vi "Get Test.vi"(8 "error in (no error)":errorcluster, 10 "Unique ID":string, 11 "Test Executive Ref":refnum<data-value>) -> (0 "error out":errorcluster, 1 "Found?":bool, 2 "Test":refnum<class "Executioner.lvclass">, 3 "Test Executive Ref out":refnum<data-value>)   [LabVIEW 2017, in "Test Executive.lvlib" / "TestExecutive Ref.lvclass"]
uses:
  <vilib>/gpm_packages/@cs/test-executive/Source/Test Executive/TestExecutive Ref/TestExecutive Ref.lvclass
  <vilib>/gpm_packages/@cs/test-executive/Source/Test Executive/ITestExecutive/ITest Executive.lvclass
  <vilib>/gpm_packages/@cs/test-executive/Source/Test Executive/Executioner/Executioner.lvclass
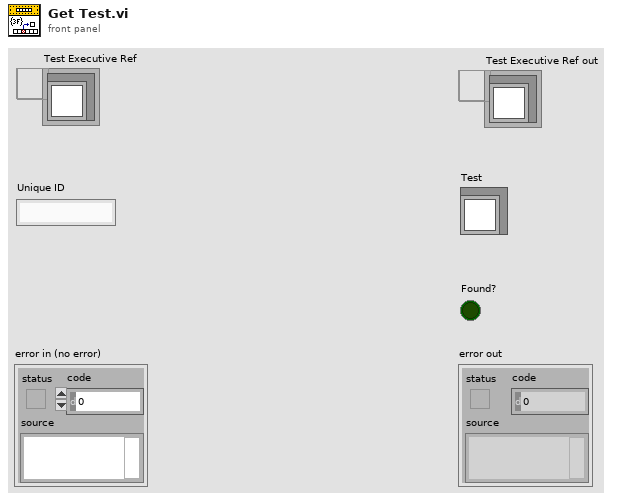
[diagram p1: front panel]
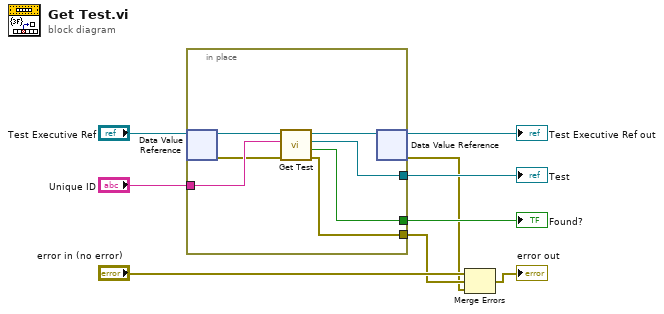
[diagram p0: block diagram]
diagram:
  n1 = in-place {
    in-place-border: [w14] -> w7
    in-place-border: [w13] -> w6
    in-place-border: "Unique ID" -> [w12]
    in-place-border: [w10] -> w3
    n2 = in-place-dvr #1("Test Executive Ref") -> (w16:refnum<class "ITest Executive.lvclass">, w11:errorcluster)
    n3 = call-dynamic "Get Test.vi"("error in (no error)"=w11, "Unique ID"=w12, "ITest Executive in"=w16) -> ("error out"=w10:errorcluster, "Found?"=w14:bool, "Test"=w13:refnum<class "Executioner.lvclass">, "ITest Executive out"=w15:refnum<class "ITest Executive.lvclass">)  [unwired: 5 in]
    n4 = in-place-dvr #1(w15) -> (→"Test Executive Ref out":refnum<data-value>, w2:errorcluster)
  }
  "Test" <- w6
  "Found?" <- w7
  n5 = Merge Errors("error in (no error)", w3, w2) -> (→"error out":errorcluster)
